vi "Write Sub Trees.vi"(8 "error in (no error)":errorcluster, 10 "Sub Trees":refnum<class "Tree.lvclass">[](array[class]), 11 "Composite Tree in":refnum<class "Composite Tree.lvclass">) -> (0 "error out":errorcluster, 3 "Composite Tree out":refnum<class "Composite Tree.lvclass">)   [LabVIEW 2019, in "Composite Tree.lvclass"]
uses:
  Composite Tree.lvclass
  Tree/Tree.lvclass
  Composite Tree.lvclass/Composite Tree.ctl
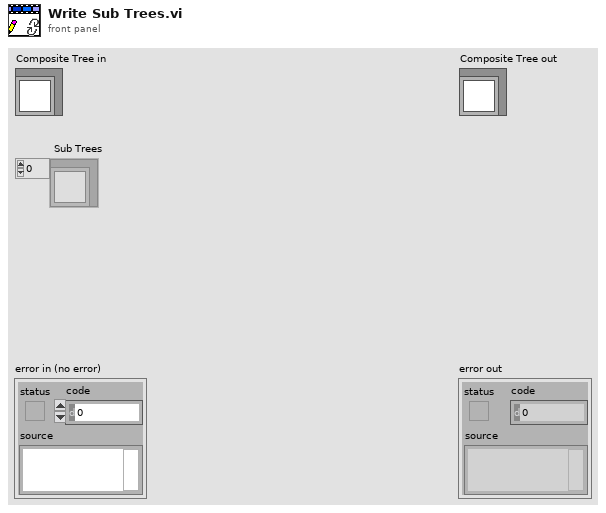
[diagram p1: front panel]
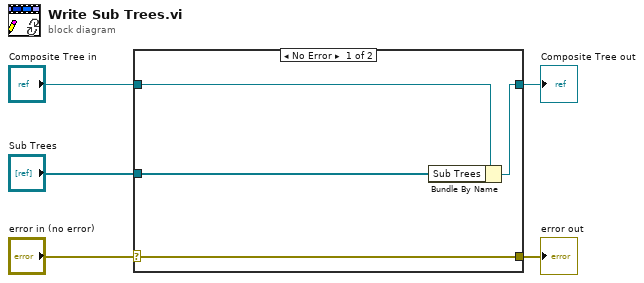
[diagram p0: block diagram]
diagram:
  n1 = case shown="No Error" "error in (no error)" {
    selector: "error in (no error)" -> [w9 w10]
    tunnel: [w9 w10] -> w4
    tunnel: [w7 w11] -> w2
    tunnel: "Composite Tree in" -> [w8 w11]
    tunnel: "Sub Trees" -> [w6 _]
    frame No Error {
      n2 = Bundle By Name(cluster=w8, "Sub Trees"=w6) -> (w7:refnum<class "Composite Tree.lvclass">)
    }
    frame Error {
    }
  }
  "error out" <- w4
  "Composite Tree out" <- w2
